vi "build_PWM_task_y.vi"(8 "error in":errorcluster) -> (0 "error out":errorcluster, 3 "task out":refnum<k21>)   [LabVIEW 2013]
uses:
  <vilib>/DAQmx/create/channels.llb/DAQmx Create Channel (CO-Pulse Generation-Time).vi
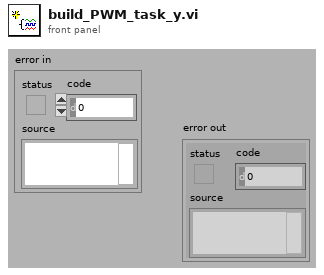
[diagram p1: front panel]
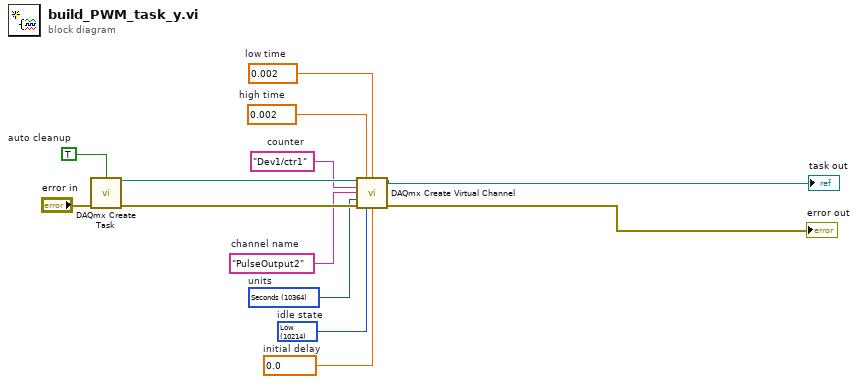
[diagram p0: block diagram]
diagram:
  w3 = 0.002  # low time
  w4 = 0.002  # high time
  w5 = 0.0  # initial delay
  w6 = 10214 items=["High"=10192, "Low"=10214]  # idle state
  w7 = 10364 items=["Seconds"=10364, "From Custom Scale"=10065]  # units
  w8 = "PulseOutput2"  # channel name
  w9 = "Dev1/ctr1"  # counter
  w11 = TRUE  # auto cleanup
  n1 = call <vilib>:"DAQmx Create Task.vi"("auto cleanup"=w11, "error in"="error in") -> ("task out"=w10:refnum<k21>, "error out"=w12:errorcluster)  [unwired: 12 in]
  n2 = call-poly <vilib>:"DAQmx Create Virtual Channel.vi"("task in"=w10, "high time"=w4, "low time"=w3, "counter"=w9, "name to assign"=w8, "units"=w7, "error in"=w12, "idle state"=w6, "initial delay"=w5) -> ("task out"=→"task out":refnum<k21>, "error out"=→"error out":errorcluster)  [unwired: 5 in]
